vi "DBTester2.vi"() -> ()   [LabVIEW 2015]
uses:
  BERTTA.dll
panel:
  out "values":dbl[](array[numeric])
  in  "col":i32=4
  in  "nrows":i32=20
  out "Mettler":dynamicdata(graph)
  in  "Device port":i32=6
  out "Weight":dbl
  out "Weight 2":dbl
  in  "Device port 2":i32=2
  out "rc":i32
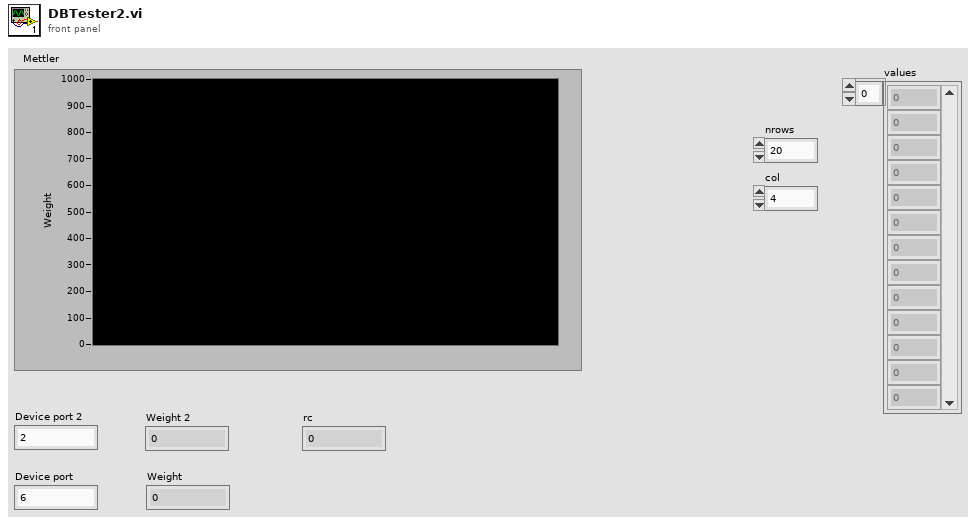
[diagram p1: front panel]
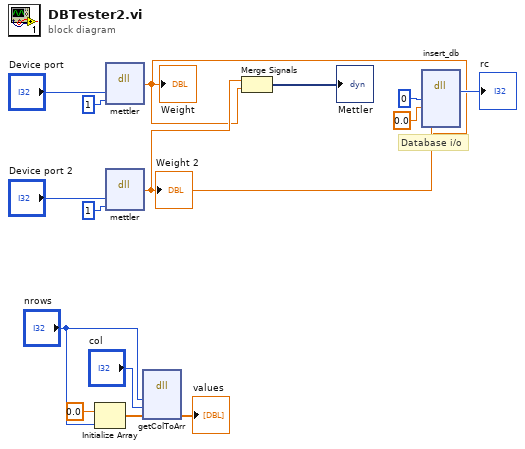
[diagram p0: block diagram]
diagram:
  # "Database i/o"
  n1 = Initialize Array(0.0 ("element"), "nrows") -> (w3:dbl[])
  n2 = dll-call lib="C:/Users/xlaraser/Documents/Visual Studio 2017/Projects/Bertta/BERTTA/Debug/BERTTA.dll" fn="mettler"("port"="Device port", "msg"=1) -> ("return type"=w8:dbl)  [unwired: 5 in, 2 out]
  "Weight" <- w8
  n3 = dll-call lib="C:/Users/xlaraser/Documents/Visual Studio 2017/Projects/Bertta/BERTTA/Debug/BERTTA.dll" fn="mettler"("port"="Device port 2", "msg"=1) -> ("return type"=w9:dbl)  [unwired: 5 in, 2 out]
  "Weight 2" <- w9
  n4 = dll-call lib="C:/Users/xlaraser/Documents/Visual Studio 2017/Projects/Bertta/BERTTA/Debug/BERTTA.dll" fn="getColToArr"("nrows"="nrows", "col"="col", "values"=w3) -> ("values"=→"values":dbl[])  [unwired: 6 in, 2 out]
  n5 = Merge Signals(w9, w8) -> (→"Mettler":dynamicdata)
  n6 = dll-call lib="C:/Users/xlaraser/Documents/Visual Studio 2017/Projects/Bertta/BERTTA/Debug/BERTTA.dll" fn="insert_db"("heidolph"=0, "lauda"=0.0, "mettler1"=w9, "mettler2"=w8) -> ("return type"=→"rc":i32)  [unwired: 7 in, 2 out]
